vi "MAV_CMD_COMPONENT_ARM_DISARM.vi"(10 "Target System and Target Component":u8=1, 11 "ARM(T)/DISARM(F)":bool) -> (3 "MAVLink Message":u8[](array[numeric]))   [LabVIEW 2014]
panel:
  out "Payload Size":i32
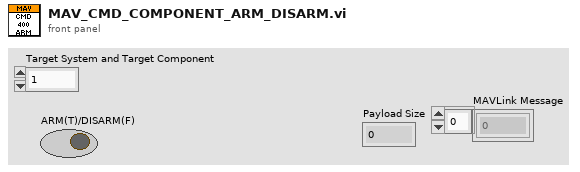
[diagram p1: front panel]
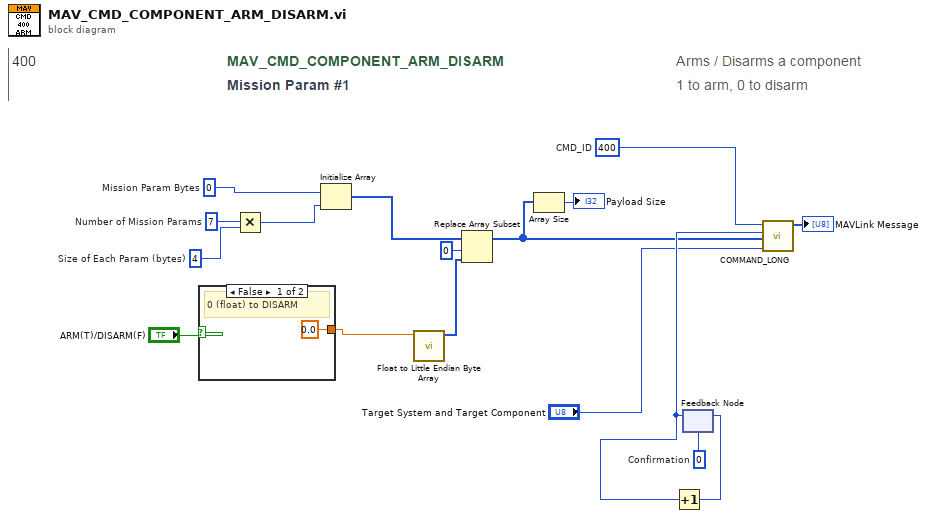
[diagram p0: block diagram]
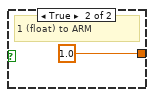
[diagram p2: hidden frame]
diagram:
  w10 = u8 0  # Confirmation
  w15 = 4  # Size of Each Param (bytes)
  w16 = 7  # Number of Mission Params
  w17 = u8 0  # Mission Param Bytes
  w5 = u16 400  # CMD_ID
  n1 = case shown="False" "ARM(T)/DISARM(F)" {
    tunnel: [sgl 0.0 sgl 1.0] -> w7
    frame False {
      # "0 (float) to DISARM"
    }
    frame True {
      # "1 (float) to ARM"
    }
  }
  n2 = Multiply(x=w16, y=w15) -> (x*y=w14:i32)
  n3 = Initialize Array(w17, w14) -> (w13:u8[])
  n4 = call "Float to Little Endian Byte Array.vi"("Float In"=w7) -> ("LE Byte Array"=w6:u8[])  [unwired: 10 in]
  n5 = Replace Array Subset(array=w13, new element=w6, index=0) -> (w3:u8[])
  n6 = Array Size(array=w3) -> (size(s)=→"Payload Size":i32)
  n7 = feedback #1(w10) -> (w4:u8)
  n8 = Increment(x=w4) -> (x+1=w9:u8)
  n9 = feedback-in #1(w9) -> ()
  n10 = call "COMMAND_LONG.vi"("Target System and Target Component"="Target System and Target Component", "Mission Params"=w3, "Confirmation"=w4, "Command ID"=w5) -> ("MAVLink Message"=→"MAVLink Message":u8[])  [unwired: 7 in]
